vi "Fit Model to Plot Core.vi"(0 "Fit Plot Information":T6={"XY Graph Ref"=refnum, "Mouse Coordinates"={"X"=0.0, "Y"=0.0}, "Fit Model"=enum."Select a Fit Model...", "Plot Index"=-1}, 1 "LM Function & Gradient":refnum<vi>, 2 "Display Plots (T)":bool=TRUE, 5 "Fit Settings":T2={"Use Original Plot # Points"=FALSE, "# Fit Plot Points"=0, "Fit Method"=0, "Weighted Fit"=FALSE, "Show All Fit Components"=FALSE, "Axis Type"=0, "Show Fit Residuals"=TRUE, "Residual Type"=enum."Standard"} {"Axis Type" items=["Linear", "Logarithmic"]; "Fit Method" items=["Least Square", "Least Absolute Residual", "Bisquare"]}, 7 "termination":cluster{"max iteration":i32, "tolerance":dbl}={"max iteration"=2000, "tolerance"=1e-08}, 9 "Additional Data (in)":variant, 11 "error in (no error)":errorcluster, 12 "Send Graph to Notebook?":bool) -> (3 "Plot Name":string, 4 "Array of Plots (Fit, Components, Residuals)":cluster{"X Array":dbl[], "Y Array":dbl[]}[](array[cluster]), 6 "best nonlinear fit":dbl[](array[numeric]), 8 "Fit Parameters Cluster":variant, 10 "Fit Parameters Uncertainties Cluster":variant, 13 "Additional Data (out)":variant, 14 "Fit Algorithm":T1, 15 "error out":errorcluster)   [LabVIEW 2019]
uses:
  Fit Plot Request Information.ctl
  <vilib>/Utility/miscctls.llb/LVPointDoubleTypeDef.ctl
  Fit Models.ctl
  Fit Settings.ctl
  <vilib>/Analysis/6fits.llb/Curve Fitting Criteria.ctl
  Calc/Ramp Type.ctl
  Residual Type.ctl
  Fit Algorithm.ctl
  Graphs/LabVIEW Plot Interpolation.ctl
  Notebook/Notebook.lvlib
  <vilib>/Analysis/NI_AALPro.lvlib
panel:
  out "Fitted Plot":cluster{"X Array":dbl[], "Y Array":dbl[]}
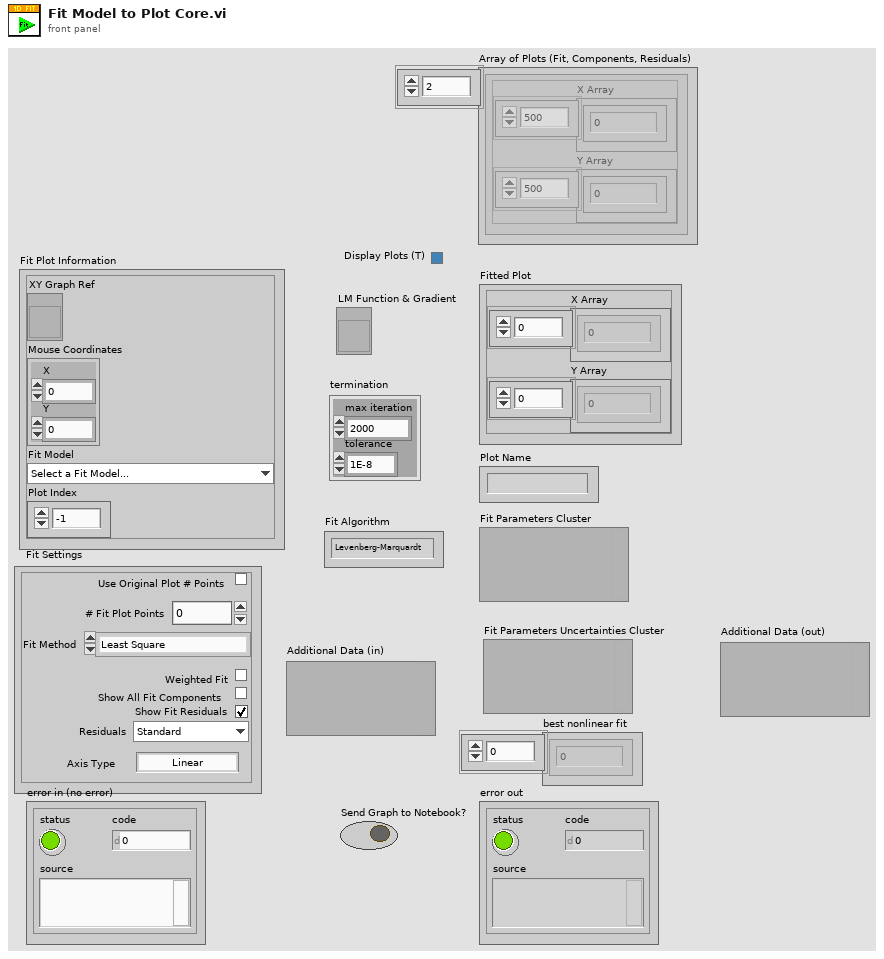
[diagram p1: front panel]
types:
  T1 = typedef "Fit Algorithm.ctl" = enum16{"Levenberg-Marquardt", "Trust-Region Dogleg"}
  T2 = typedef "Fit Settings.ctl" = cluster{"Use Original Plot # Points":bool, "# Fit Plot Points":u32, "Fit Method":T3, "Weighted Fit":bool, "Show All Fit Components":bool, "Axis Type":T4, "Show Fit Residuals":bool, "Residual Type":T5}
  T3 = typedef "NI_AALPro.lvlib/Curve Fitting Criteria.ctl" = u16
  T4 = typedef "Ramp Type.ctl" = u16
  T5 = typedef "Residual Type.ctl" = enum16{"Standard", "Normalized", "Reduced"}
  T6 = typedef "Fit Plot Request Information.ctl" = cluster{"XY Graph Ref":refnum<vi>, "Mouse Coordinates":T7, "Fit Model":T8, "Plot Index":i32}
  T7 = typedef "LVPointDoubleTypeDef.ctl" = cluster{"X":dbl, "Y":dbl}
  T8 = typedef "Fit Models.ctl" = enum16{"Select a Fit Model...", "           Single Peak", "Gaussian", "Asymmetric Gaussian", "Lorentzian", "Asymmetric Lorentzian", "Gaussian/Lorentzian", "Lorentzian/Gaussian", "           Double Peak", "Two Gaussians", "Two Asymmetric Gaussians", "Two H-Connected Gaussians", "Two T-Connected Gaussians", "Two H-Connected Asymmetric Gaussians", "Two T-Connected Asymmetric Gaussians", "           Triple Peak", "Three Gaussians", "Three Asymmetric Gaussians", "              Decays", "1-Exponential", "IRF*PSED", "2-Exponentials", "               ACF", "2D Gaussian ACF", "2D Gaussian + Blinking ACF", "2D Gaussian + Flow ACF", "3D Gaussian ACF", "3D Gaussian + Blinking ACF", "             Multiplot", "2D Gaussian ACF & 2D Gaussian + Flow ACF"}
  T9 = typedef "XY Plot Data.ctl" = cluster{"X Array":dbl[], "Y Array":dbl[]}
  T10 = cluster{"X Array":dbl[], "Y Array":dbl[], "Weights":dbl[]}
  T11 = cluster{"parameter minimum":dbl[], "parameter maximum":dbl[]}
  T12 = typedef "Fit Statistics.ctl" = cluster{"# iterations":i32, "number of function calls":i32, "chi2":dbl, "residue":dbl}
  T13 = cluster{"best fit parameters":dbl[], "best nonlinear fit":dbl[]}
  T14 = typedef "LabVIEW Plot Interpolation.ctl" = u8
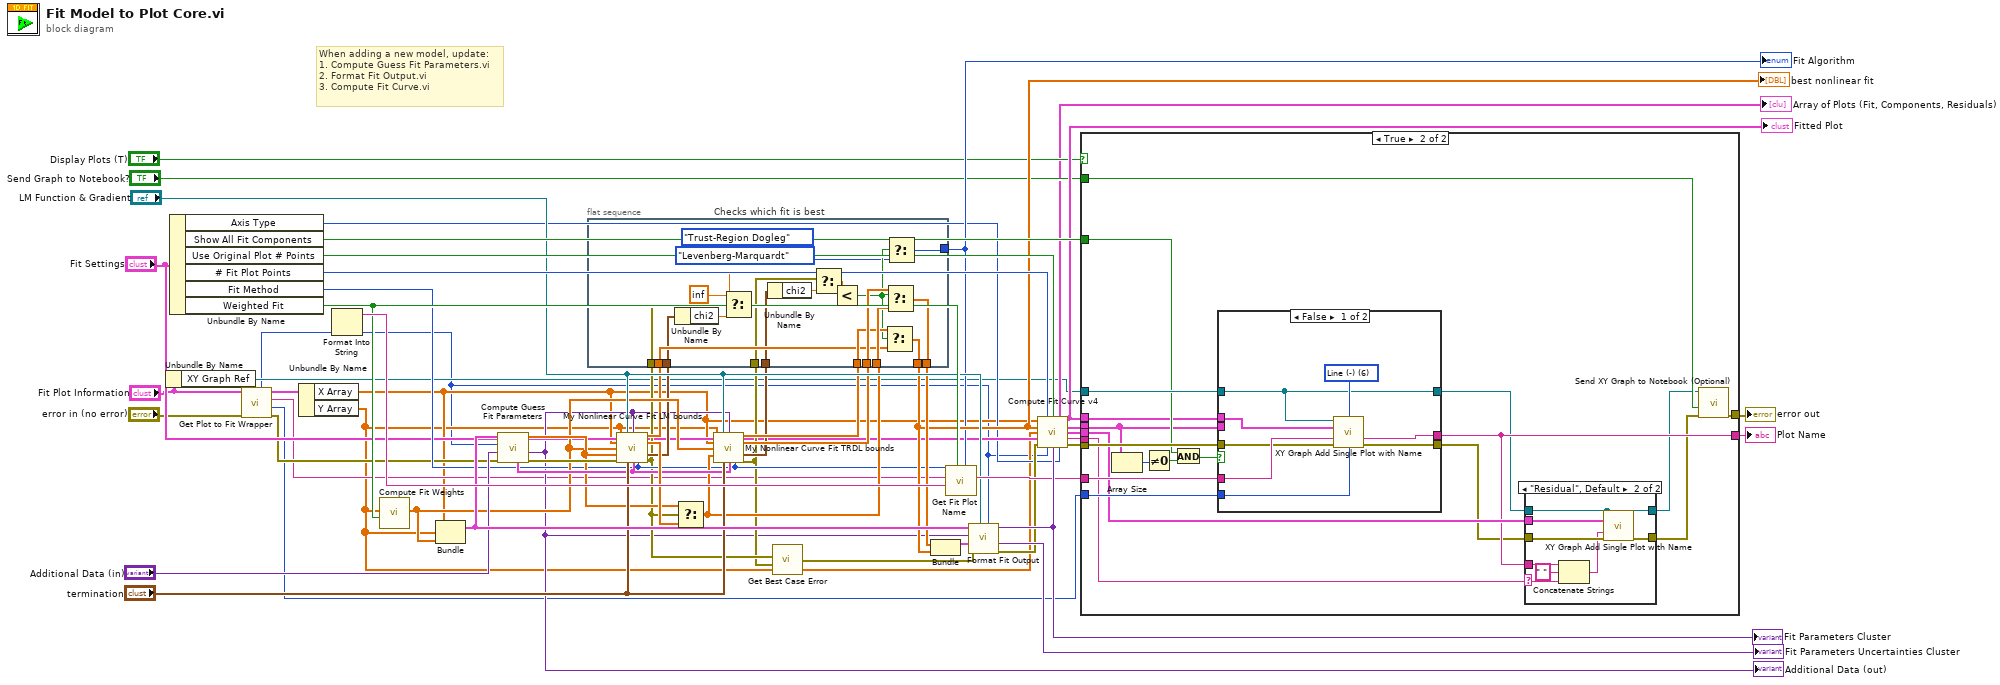
[diagram p0: block diagram]
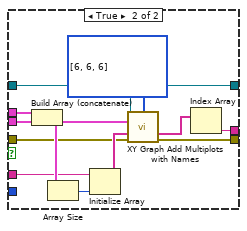
[diagram p4: hidden frame]
diagram:
  # "When adding a new model, update:\n1. Compute Guess Fit Parameters.vi\n2. Format Fit Output.vi\n3. Compute Fit Curve.vi"
  n1 = Unbundle By Name("Fit Plot Information") -> ("XY Graph Ref"=w7:refnum<vi>)
  n2 = Unbundle By Name("Fit Settings") -> ("Axis Type"=w13:T4, "Show All Fit Components"=w42:bool, "Use Original Plot # Points"=w52:bool, "# Fit Plot Points"=w53:u32, "Fit Method"=w26:T3, "Weighted Fit"=w54:bool)
  n3 = call "Get Plot to Fit Wrapper.vi"("error in (no error)"="error in (no error)", "Fit Plot Information"="Fit Plot Information") -> ("error out"=w8:errorcluster, "Plot Color"=w6:u32, "Plot Name"=w5:string, "Plot"=w4:T9, "Fit Model"=w1:T8)  [unwired: 5 in]
  n4 = Unbundle By Name(w4) -> ("X Array"=w3:dbl[], "Y Array"=w2:dbl[])
  n5 = Format Into String(w1) -> (resulting string=w55:string)  [unwired: 3 in, 1 out]
  n6 = call "Compute Fit Weights.vi"("Use Weights? (F)"=w54, "Function Values"=w2) -> ("Weights"=w34:dbl[])  [unwired: 9 in]
  n7 = Bundle("X Array"=w3, "Y Array"=w2, "Weights"=w34) -> (w50:T10)  [unwired: 1 in]
  n8 = call "Compute Guess Fit Parameters.vi"("error in (no error)"=w8, "Additional Data"="Additional Data (in)", "Fit Model"=w1, "Data in"=w50) -> ("error out"=w45:errorcluster, "Additional LM Data"=w11:variant, "Initial Fit Parameters"=w35:dbl[], "Parameter Bounds"=w37:T11)  [unwired: 4 in]
  "Additional Data (out)" <- w11
  n9 = flat-sequence "Checks which fit is best" {
    tunnel: w32 -> [w74]
    tunnel: w31 -> [w73]
    tunnel: [w72] -> w30
    tunnel: w29 -> [w71]
    tunnel: w28 -> [w70]
    tunnel: [w69] -> w27
    tunnel: [w65] -> w25
    tunnel: w23 -> [w64]
    tunnel: w24 -> [w63]
    tunnel: w22 -> [w61]
    tunnel: w21 -> [w57]
    frame #0 {
      w56 = inf ("t")
      n10 = Unbundle By Name(w63) -> ("chi2"=w62:dbl)
      n11 = Select(t=w56, s=w61, f=w62) -> (s? t:f=w60:dbl)
      n12 = Unbundle By Name(w64) -> ("chi2"=w59:dbl)
      n13 = Select(t=w56, s=w57, f=w59) -> (s? t:f=w58:dbl)
      n14 = Less?(x=w58, y=w60) -> (x < y?=w68:bool)
      n15 = Select(t=w71, s=w68, f=w70) -> (s? t:f=w69:dbl[])
      n16 = Select(t=w74, s=w68, f=w73) -> (s? t:f=w72:dbl[])
      n17 = Select(t=Fit_Algorithm."Trust-Region Dogleg" ("Fit Algorithm"), s=w68, f=Fit_Algorithm."Levenberg-Marquardt" ("Fit Algorithm")) -> (s? t:f=w65:T1)
    }
  }
  n18 = call "My Nonlinear Curve Fit LM bounds.vi"("Y"=w2, "f(x,a)"="LM Function & Gradient", "data"=w11, "X"=w3, "Weight"=w34, "initial parameters"=w35, "error in (no error)"=w45, "termination"="termination", "parameter bounds"=w37, "method"=w26) -> ("best nonlinear fit"=w28:dbl[], "best fit parameters"=w38:dbl[], "Fit Statistics"=w24:T12, "error out"=w22:errorcluster)  [unwired: 2 out]
  n19 = Select(t=w35, s=w22, f=w38) -> (s? t:f=w31:dbl[])
  n20 = call "My Nonlinear Curve Fit TRDL bounds.vi"("Y"=w2, "f(x,a)"="LM Function & Gradient", "data"=w11, "X"=w3, "Weight"=w34, "initial parameters"=w31, "termination"="termination", "parameter bounds"=w37, "method"=w26) -> ("best nonlinear fit"=w29:dbl[], "best fit parameters"=w32:dbl[], "Fit Statistics"=w23:T12, "error out"=w21:errorcluster)  [unwired: 1 in, 2 out]
  n21 = call "Get Best Case Error.vi"("error 2 in (no error)"=w21, "error 1 in (no error)"=w22) -> ("error out"=w33:errorcluster)  [unwired: 4 in]
  n22 = Bundle("best fit parameters"=w30, "best nonlinear fit"=w27) -> (w48:T13)  [unwired: 1 in]
  n23 = call "Get Fit Plot Name.vi"("Fit Algorithm"=w25, "Weighted Histogram Fit"=w54, "Fit Model"=w55, "Plot Name"=w5, "Fit Method"=w26) -> ("Fit Plot Name"=w47:string)  [unwired: 6 in]
  n24 = call "Format Fit Output.vi"("Fit Model"=w1, "f(x,a)"="LM Function & Gradient", "Error In"=w33, "Fit Results"=w48, "Additional Data"=w11, "Data in"=w50) -> ("Error Out"=w44:errorcluster, "Fit Parameters Uncertainties Cluster"=→"Fit Parameters Uncertainties Cluster":variant, "Fit Parameters Cluster"=w51:variant)  [unwired: 3 in]
  "Fit Parameters Cluster" <- w51
  n25 = call "Compute Fit Curve v4.vi"("X Array in"=w3, "# Points"=w53, "Use Same Number of Points as Histogram"=w52, "Best Fit in"=w27, "Y Array in"=w2, "Fit Settings"="Fit Settings", "Error In"=w44, "Fit Model"=w1, "Fit Parameters"=w51, "Ramp Type"=w13) -> ("Array of Plots (Fit, Components, Residuals)"=→"Array of Plots (Fit, Components, Residuals)":cluster{"X Array":dbl[], "Y Array":dbl[]}[], "Fitted Plot"=w41:cluster{"X Array":dbl[], "Y Array":dbl[]}, "Array of Component Plots"=w40:cluster{"X Array":dbl[], "Y Array":dbl[]}[], "Residual Plot"=w16:cluster{"X Array":dbl[], "Y Array":dbl[]}, "Residual Type"=w17:string, "Error Out"=w46:errorcluster)
  "Fitted Plot" <- w41
  n26 = case shown="True" "Display Plots (T)" {
    tunnel: w47 -> [w75 w95]
    tunnel: w6 -> [_ w94]
    tunnel: w46 -> [w76 w93]
    tunnel: w7 -> [_ w92]
    tunnel: w42 -> [_ w89]
    tunnel: w41 -> [_ w87]
    tunnel: w40 -> [_ w86]
    tunnel: "Send Graph to Notebook?" -> [_ w85]
    tunnel: [w76 w84] -> w19
    tunnel: w17 -> [_ w83]
    tunnel: w16 -> [_ w82]
    tunnel: [w75 w81] -> w15
    frame False {
    }
    frame True {
      n27 = Array Size(array=w86) -> (size(s)=w91:i32)
      n28 = Not Equal To 0?(x=w91) -> (x != 0?=w90:bool)
      n29 = And(x=w89, y=w90) -> (x .and. y?=w88:bool)
      n30 = case shown="False" w88 {
        tunnel: w95 -> [w113 w114]
        tunnel: [w111 w117] -> w80
        tunnel: [w110 w116] -> w81
        tunnel: w94 -> [w109 _]
        tunnel: w93 -> [w108 w118]
        tunnel: w92 -> [w106 w115]
        tunnel: w87 -> [w107 w120]
        tunnel: w86 -> [_ w119]
        tunnel: [w106 w115] -> w78
        frame False {
          w112 = T14 6 items=["Point (.)", "Stepwise Right (--.)", "Stepwise Centered (-.-)", "Line + Point (\\. /)", "Stepwise Left (.--)", "Stepwise Vertical (|.|)", "Line (-)", "Use Previous Plot's Style"] ("Plot Interpolation (Previous Plot's Style)")
          n31 = call "XY Graph Add Single Plot with Name.vi"("XYGraph Ref in"=w106, "Plot Interpolation (Previous Plot's Style)"=w112, "Plot"=w107, "Plot Name (\"Plot\")"=w113, "error in (no error)"=w108, "Plot Color (Default)"=w109) -> ("Plot Name"=w110:string, "error out"=w111:errorcluster)  [unwired: 6 in, 2 out]
        }
        frame True {
          w121 = T14[] [6, 6, 6] items=["Point (.)", "Stepwise Right (--.)", "Stepwise Centered (-.-)", "Line + Point (\\. /)", "Stepwise Left (.--)", "Stepwise Vertical (|.|)", "Line (-)", "Use Previous Plot's Style"] ("Plots Interpolation (Previous Plot's Style)")
          n32 = Build Array (concatenate)(w120, w119) -> (w125:cluster{"X Array":dbl[], "Y Array":dbl[]}[])
          n33 = Array Size(array=w125) -> (size(s)=w124:i32)
          n34 = Initialize Array(w114, w124) -> (w123:string[])
          n35 = call "XY Graph Add Multiplots with Names.vi"("XYGraph in"=w115, "Plots Interpolation (Previous Plot's Style)"=w121, "Array of Plots"=w125, "Array of Plot Names (\"Plot\")"=w123, "error in (no error)"=w118) -> ("Added Plot Names"=w122:string[], "error out"=w117:errorcluster)  [unwired: 6 in, 3 out]
          n36 = Index Array(array=w122) -> (element=w116:string)  [unwired: 1 in]
        }
      }
      n37 = case shown="\"Residual\", Default" w83 {
        selector: w83 -> [_ w100]
        tunnel: w82 -> [_ w104]
        tunnel: w81 -> [_ w101]
        tunnel: w78 -> [w97 w102]
        tunnel: w80 -> [w96 w105]
        tunnel: [w96 w103] -> w79
        tunnel: [w97 w102] -> w77
        frame "" {
        }
        frame "Residual", Default {
          n38 = Concatenate Strings(w101, " " ("string"), w100) -> (w98:string)
          n39 = call "XY Graph Add Single Plot with Name.vi"("XYGraph Ref in"=w102, "Plot"=w104, "Plot Name (\"Plot\")"=w98, "error in (no error)"=w105) -> ("error out"=w103:errorcluster)  [unwired: 8 in, 3 out]
        }
      }
      n40 = call "Send XY Graph to Notebook (Optional).vi"("error in (no error)"=w79, "Send Graph to Notebook?"=w85, "XYGraph in"=w77) -> ("error out"=w84:errorcluster)  [unwired: 8 in]
    }
  }
  "error out" <- w19
  "Plot Name" <- w15
  "Fit Algorithm" <- w25
  "best nonlinear fit" <- w27
